vi "PV CHECKSUM_256.VI"(1 "input string":string) -> (0 "checksum":string)   [LabVIEW 2024, in "Pfeiffer Vacuum.lvlib"]
uses:
  <instrlib>/Pfeiffer Vacuum/Pfeiffer Vacuum.lvlib
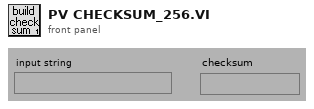
[diagram p1: front panel]
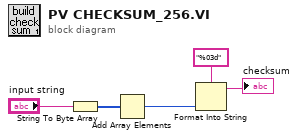
[diagram p0: block diagram]
diagram:
  n1 = String To Byte Array(string="input string") -> (unsigned byte array=w2:u8[])
  n2 = Add Array Elements(numeric array=w2) -> (sum=w1:u8)
  n3 = Format Into String(format string="%03d" ("Format-String"), w1) -> (resulting string=→"checksum":string)  [unwired: 2 in, 1 out]
